vi "Main.vi"(5 "Deliminated Char":string=".", 6 "PLC Folder names":string[](array[string])=["StaARx#[PLC]StaATesterRxSignals", "StaATx#[PLC]StaATesterTxSignals"], 7 "PLC FGVname":string="OPC Ref", 8 "error in":errorcluster, 9 "Sequence Context In":refnum<k7>, 10 "Event Sources":T1, 11 "PostUUT In":refnum<class "PostUUT.lvclass">) -> (0 "error out":errorcluster, 2 "Station":string, 3 "OPC UA Out":refnum<class "PostUUT.lvclass">)   [LabVIEW 2021, in "OPC UA.lvlib" / "PostUUT.lvclass"]
uses:
  PostUUT.lvclass
  Controls/Rx PostUUT.ctl
  Controls/Tx PostUUT.ctl
  PostUUT.lvclass/PostUUT.ctl
  <vilib>/addons/TestStand/_TSUtility.llb/TestStand - Get Property Value (Number {Signed 32-bit Integer}).vi
  OPC UA/OPC UA.lvclass
panel:
  out "Connect?":bool
  in  "Tx Tester":T2={"ResultsReady"=TRUE, "Results"=0, "ElapsedTime"=0, "TimeCompleted"=[], "Fault"=FALSE, "Timeout"=FALSE, "Heartbeat"=FALSE}
  out "Rx PostUUT":T3
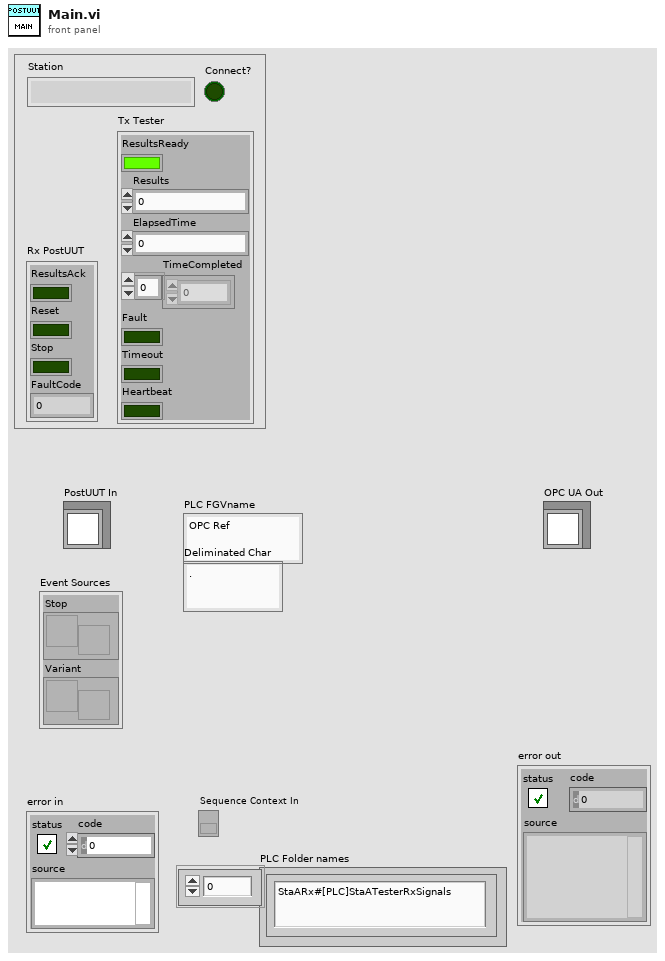
[diagram p1: front panel]
types:
  T1 = cluster{"Stop":refnum<user-event>, "Variant":refnum<user-event>}
  T2 = typedef "OPC UA.lvlib/PostUUT.lvclass/Tx PostUUT.ctl" = cluster{"ResultsReady":bool, "Results":u32, "ElapsedTime":i32, "TimeCompleted":i32[], "Fault":bool, "Timeout":bool, "Heartbeat":bool}
  T3 = typedef "OPC UA.lvlib/PostUUT.lvclass/Rx PostUUT.ctl" = cluster{"ResultsAck":bool, "Reset":bool, "Stop":bool, "FaultCode":u32}
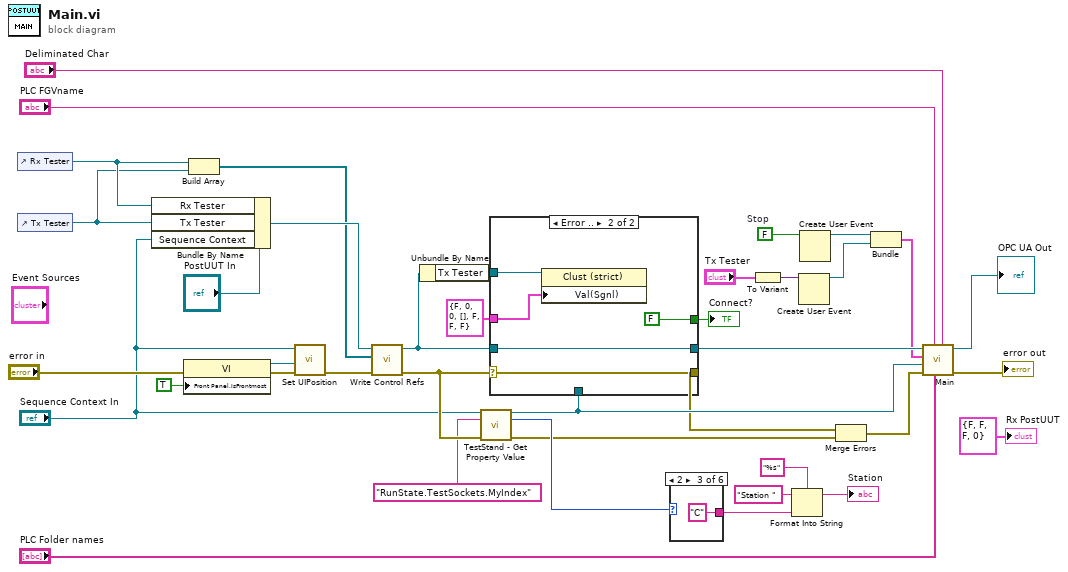
[diagram p0: block diagram]
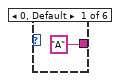
[diagram p2: hidden frame]
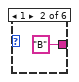
[diagram p3: hidden frame]
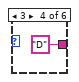
[diagram p4: hidden frame]
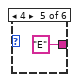
[diagram p5: hidden frame]
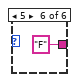
[diagram p6: hidden frame]
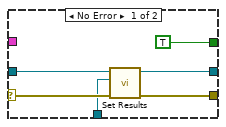
[diagram p7: hidden frame]
diagram:
  w25 = FALSE  # Stop
  n1 = control-ref of="Rx Tester"() -> (w33:refnum<vi>)
  n2 = control-ref of="Tx Tester"() -> (w32:refnum<vi>)
  n3 = Bundle By Name(cluster="PostUUT In", "Rx Tester"=w33, "Tx Tester"=w32, "Sequence Context"="Sequence Context In") -> (w31:refnum<class "PostUUT.lvclass">)
  n4 = property class="VI"(error in="error in", "Front Panel.IsFrontmost"=TRUE ("Front Panel Window:Is Frontmost")) -> (reference out=w18:refnum<vi>, error out=w20:errorcluster)  [unwired: 1 in]
  n5 = Build Array(w33, w32) -> (w30:refnum<vi>[])
  n6 = call "Set UIPosition.vi"("error in"=w20, "VI Ref"=w18, "Sequence Context In"="Sequence Context In") -> ("error out"=w19:errorcluster)  [unwired: 8 in]
  n7 = call-dynamic "Write Control Refs.vi"("error in (no error)"=w19, "Ctl Refs"=w30, "OPC UA in"=w31) -> ("error out"=w6:errorcluster, "OPC UA out"=w27:refnum<class "PostUUT.lvclass">)  [unwired: 7 in]
  n8 = Unbundle By Name(w27) -> ("Tx Tester"=w35:refnum<vi>)
  n9 = call-poly <vilib>:"TestStand - Get Property Value.vi"("Sequence Context In"="Sequence Context In", "Lookup String"="RunState.TestSockets.MyIndex", "error in (no error)"=w6) -> ("Sequence Context Out"=w3:refnum<k7>, "Value"=w12:i32, "error out"=w7:errorcluster)  [unwired: 10 in]
  n10 = case shown="Error .." w6 {
    selector: w6 -> [w43 w46]
    tunnel: w27 -> [w45 w50]
    tunnel: [w40 w50] -> w23
    tunnel: w35 -> [_ w49]
    tunnel: T2 {"ResultsReady"=FALSE, "Results"=0, "ElapsedTime"=0, "TimeCompleted"=[], "Fault"=FALSE, "Timeout"=FALSE, "Heartbeat"=FALSE} ("Value (Signaling)") -> [_ w48]
    tunnel: [TRUE ("Connect?") FALSE ("Connect?")] -> w15
    tunnel: [w41 w46] -> w1
    tunnel: w3 -> [w42 _]
    frame No Error {
      n11 = call "Set Results.vi"("error in (no error)"=w43, "Sequence Context"=w42, "PostUUT in"=w45) -> ("error out"=w41:errorcluster, "PostUUT out"=w40:refnum<class "PostUUT.lvclass">)  [unwired: 7 in]
    }
    frame Error {
      n12 = property class="Clust (strict)"(reference=w49, "Val(Sgnl)"=w48) -> ()  [unwired: 1 in, 2 out]
    }
  }
  "Connect?" <- w15
  n13 = case shown="2" w12 {
    tunnel: ["A" ("format string") "B" ("format string") "C" ("format string") "D" ("format string") "E" ("format string") "F" ("format string")] -> w13
    frame 0, Default {
    }
    frame 1 {
    }
    frame 2 {
    }
    frame 3 {
    }
    frame 4 {
    }
    frame 5 {
    }
  }
  n14 = To Variant(anything="Tx Tester") -> (Variant=w38:variant)
  n15 = Format Into String(format string="%s", initial string="Station ", w13) -> (resulting string=→"Station":string)  [unwired: 1 in, 1 out]
  n16 = Create User Event(user event datatype=w38) -> (user event=w24:refnum<user-event>)  [unwired: 1 in, 1 out]
  n17 = Create User Event(user event datatype=w25) -> (user event=w26:refnum<user-event>)  [unwired: 1 in, 1 out]
  n18 = Merge Errors(w1, w7) -> (w2:errorcluster)
  n19 = Bundle("Stop"=w26, "Variant"=w24) -> (w16:T1)  [unwired: 1 in]
  n20 = call-parent "Main.vi"("Deliminated Char"="Deliminated Char", "Folder names"="PLC Folder names", "FGVname"="PLC FGVname", "error in"=w2, "Sequence Context In"=w3, "Event Sources"=w16, "OPC UA In"=w23) -> ("error out"=→"error out":errorcluster, "OPC UA Out"=→"OPC UA Out":refnum<class "PostUUT.lvclass">)  [unwired: 2 in, 1 out]
  "Rx PostUUT" <- T3 {"ResultsAck"=FALSE, "Reset"=FALSE, "Stop"=FALSE, "FaultCode"=0} ("Rx PostUUT")
